vi "打开通讯连接.vi"(11 "簇":T1) -> ()   [LabVIEW 2017]
panel:
  out "error out":errorcluster
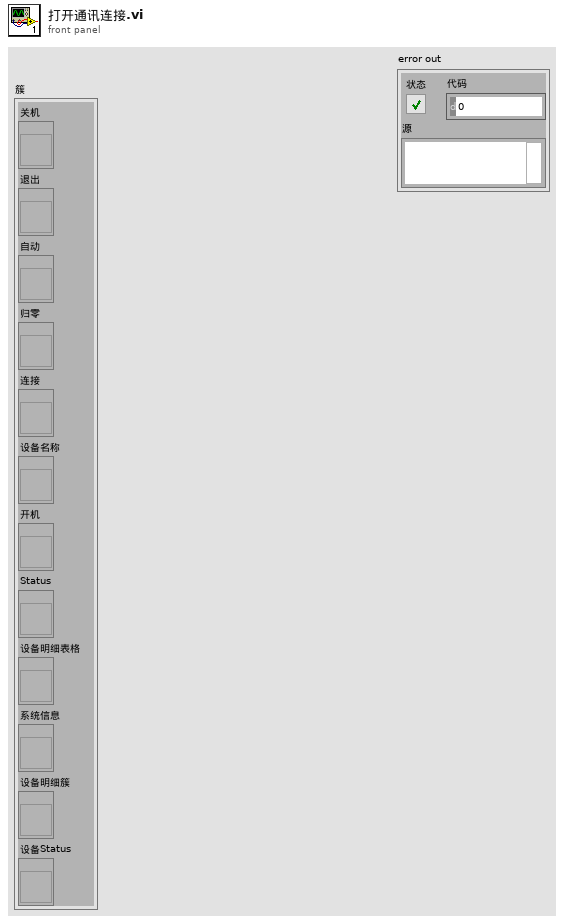
[diagram p1: front panel]
types:
  T1 = typedef "界面控件引用.ctl" = cluster{"关机":refnum<vi>, "退出":refnum<vi>, "自动":refnum<vi>, "归零":refnum<vi>, "连接":refnum<vi>, "设备名称":refnum<vi>, "开机":refnum<vi>, "Status":refnum<vi>, "设备明细表格":refnum<vi>, "系统信息":refnum<vi>, "设备明细簇":refnum<vi>, "设备Status":refnum<vi>}
  T2 = typedef "设备名称.ctl" = enum16{"1号电脑", "2号电脑"}
  T3 = typedef "单台设备明细.ctl" = cluster{"设备名称":string, "IP地址":string, "允许开机":bool, "允许连接":bool, "允许归零":bool, "允许自动":bool, "允许退出":bool, "允许关机":bool, "connection ID":refnum<k5>}
  T4 = typedef "Status.ctl" = cluster{"开机":bool, "连接":bool, "归零":bool, "自动":bool, "退出":bool, "关机":bool}
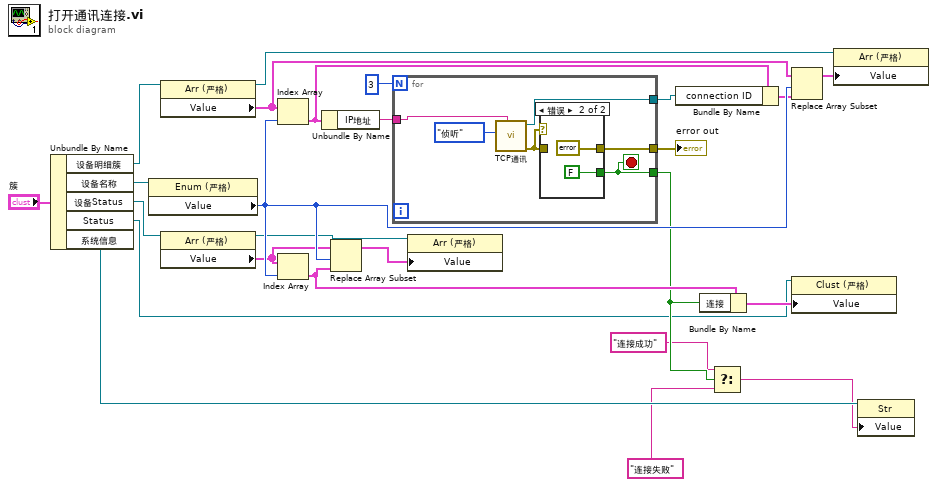
[diagram p0: block diagram]
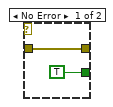
[diagram p2: hidden frame]
diagram:
  n1 = Unbundle By Name("簇") -> ("设备明细簇"=w10:refnum<vi>, "设备名称"=w11:refnum<vi>, "设备Status"=w19:refnum<vi>, "Status"=w1:refnum<vi>, "系统信息"=w5:refnum<vi>)
  n2 = property class="Enum (严格)"(reference=w11) -> ("Value"=w23:T2)  [unwired: 1 in, 2 out]
  n3 = property class="Arr (严格)"(reference=w10) -> (reference out=w13:refnum<vi>, "Value"=w15:T3[])  [unwired: 1 in, 1 out]
  n4 = property class="Arr (严格)"(reference=w19) -> (reference out=w20:refnum<vi>, "Value"=w22:T4[])  [unwired: 1 in, 1 out]
  n5 = Index Array(array=w15, index=w23) -> (element=w14:T3)
  n6 = Index Array(array=w22, index=w23) -> (element=w24:T4)
  n7 = Unbundle By Name(w14) -> ("IP地址"=w12:string)
  n8 = Replace Array Subset(array=w22, new element=w24, index=w23) -> (w25:T4[])
  n9 = for {
    N: 3 -> [_]
    tunnel: [w31] -> w18
    tunnel: w12 -> [w30]
    tunnel: [w28] -> w7
    tunnel: [w26] -> w6
    stop <- w26 stop-if-true
    n10 = call "TCP通讯.vi"("service name"=w30, "选项"=enum16{"NA", "侦听", "读取", "写入", "关闭"}."侦听") -> ("error out"=w27:errorcluster, "connection ID out"=w31:refnum<k5>)  [unwired: 5 in, 3 out]
    n11 = case shown="错误" w27 {
      tunnel: [TRUE FALSE] -> w26
      tunnel: [w32 errorcluster {"status"=FALSE, "code"=0, "source"=""} ("error out")] -> w28
      tunnel: w27 -> [w32 _]
      frame No Error {
      }
      frame Error {
      }
    }
  }
  "error out" <- w7
  n12 = property on="属性节点" class="Arr (严格)"(reference=w20, "Value"=w25) -> ()  [unwired: 1 in, 2 out]
  n13 = Bundle By Name(cluster=w14, "connection ID"=w18) -> (w16:T3)
  n14 = Bundle By Name(cluster=w24, "连接"=w6) -> (w21:T4)
  n15 = Select(t="连接成功", s=w6, f="连接失败") -> (s? t:f=w4:string)
  n16 = Replace Array Subset(array=w15, new element=w16, index=w23) -> (w17:T3[])
  n17 = property class="Clust (严格)"(reference=w1, "Value"=w21) -> ()  [unwired: 1 in, 2 out]
  n18 = property class="Arr (严格)"(reference=w13, "Value"=w17) -> ()  [unwired: 1 in, 2 out]
  n19 = property class="Str"(reference=w5, "Value"=w4) -> ()  [unwired: 1 in, 2 out]
